vi "Step4_4_LowPass.vi"(9 "s_axis_data_tdata":fxp<+/-,24,1>, 10 "s_axis_data_tvalid":bool) -> (1 "m_axis_data_tdata":fxp<+/-,24,1>, 2 "m_axis_data_tvalid":bool, 3 "s_axis_data_tready":bool)   [LabVIEW 2018]
uses:
  <vilib>/rvi/IPIntegrationNode/IPINode_Typedef/niFpgaIPINodeSupportedFamilies.ctl
  <vilib>/rvi/IPIntegrationNode/IPINode_Utilities/niFpgaIPINodeSimCore.vi
  <vilib>/rvi/XilinxIP/XIPIN_XNode/niFpgaXIPIN.xnode
  FIR_Filter_Configuration/FIR Compiler/xsim.dir/FIR_Compiler_3CE652926F5B43F18022D1349C670FA0/xsimk_3CE652926F5B43F18022D1349C670FA0.dll
  <vilib>/rvi/IPIntegrationNode/IPINode_Xnode/niFpgaIPINode.xnode
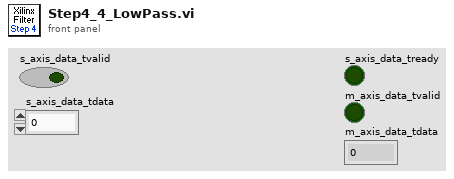
[diagram p1: front panel]
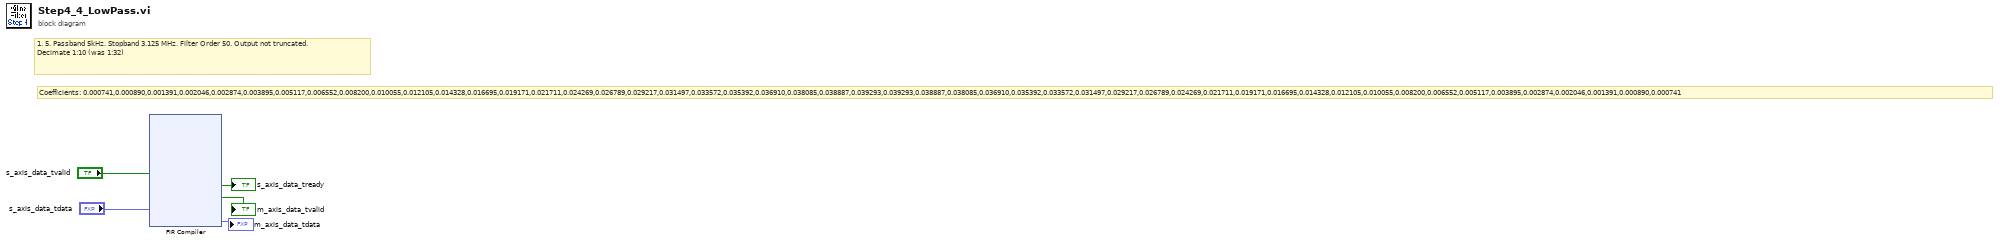
[diagram p0: block diagram]
diagram:
  # "Coefficients: 0.000741,0.000890,0.001391,0.002046,0.002874,0.003895,0.005117,0.006552,0.008200,0.010055,0.012105,0.014328,0.016695,0.019171,0.021711,0.024269,0.026789,0.029217,0.031497,0.033572,0.035392,0.036910,0.038085,0.038887,0.039293,0.039293,0.038887,0.038085,0.036910,0.035392,0.033572,0.031497,0.029217,0.026789,0.024269,0.021711,0.019171,0.016695,0.014328,0.012105,0.010055,0.008200,0.006552,0.005117,0.003895,0.002874,0.002046,0.001391,0.000890,0.000741"
  # "1.\t5.\tPassband 5kHz. Stopband 3.125 MHz. Filter Order 50. Output not truncated.\nDecimate 1:10 (was 1:32)"
  n1 = xnode ("FIR Compiler")("s_axis_data_tvalid"="s_axis_data_tvalid", "s_axis_data_tdata"="s_axis_data_tdata") -> ("s_axis_data_tready"=→"s_axis_data_tready":bool, "m_axis_data_tvalid"=→"m_axis_data_tvalid":bool, "m_axis_data_tdata"=→"m_axis_data_tdata":fxp<+/-,24,1>)
